vi "PCI-USB_ DO Notifier info.vi"(8 "error in":errorcluster, 10 "DO":T1) -> (0 "error out":errorcluster, 2 "Digital Output":bool[](array[boolean]), 3 "Update":bool)   [LabVIEW 2015]
uses:
  Digital out put.ctl
panel:
  in  "timeout in ms (-1)":i32=100
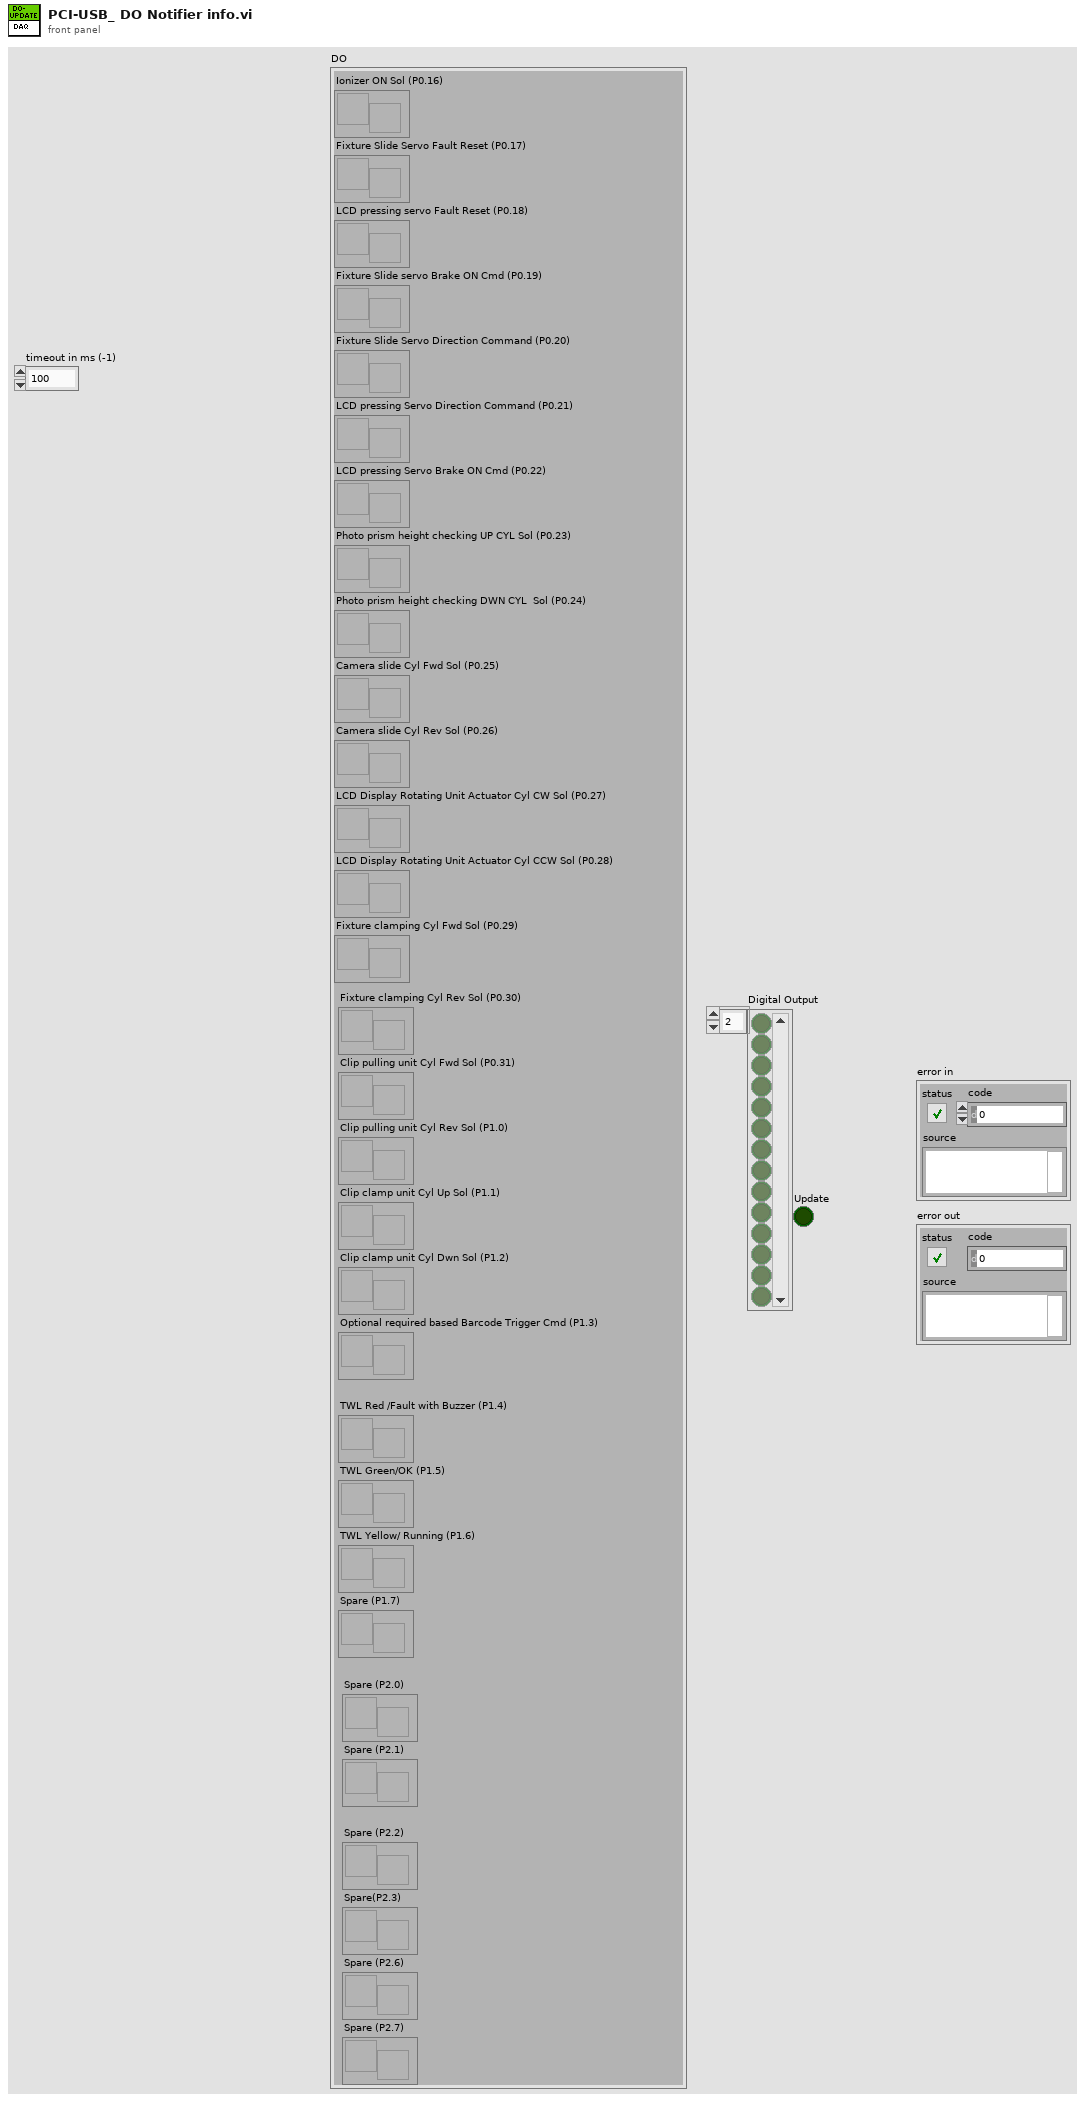
[diagram p1: front panel]
types:
  T1 = typedef "Digital out put.ctl" = cluster{"Ionizer ON Sol (P0.16)":refnum<notifier>, "Fixture Slide Servo Fault Reset (P0.17)":refnum<notifier>, "LCD pressing servo Fault Reset (P0.18)":refnum<notifier>, "Fixture Slide servo Brake ON Cmd (P0.19)":refnum<notifier>, "Fixture Slide Servo Direction Command (P0.20)":refnum<notifier>, "LCD pressing Servo Direction Command (P0.21)":refnum<notifier>, "LCD pressing Servo Brake ON Cmd (P0.22)":refnum<notifier>, "Photo prism height checking UP CYL Sol (P0.23)":refnum<notifier>, "Photo prism height checking DWN CYL  Sol (P0.24)":refnum<notifier>, "Camera slide Cyl Fwd Sol (P0.25)":refnum<notifier>, "Camera slide Cyl Rev Sol (P0.26)":refnum<notifier>, "LCD Display Rotating Unit Actuator Cyl CW Sol (P0.27)":refnum<notifier>, "LCD Display Rotating Unit Actuator Cyl CCW Sol (P0.28)":refnum<notifier>, "Fixture clamping Cyl Fwd Sol (P0.29)":refnum<notifier>, "Fixture clamping Cyl Rev Sol (P0.30)":refnum<notifier>, "Clip pulling unit Cyl Fwd Sol (P0.31)":refnum<notifier>, "Clip pulling unit Cyl Rev Sol (P1.0)":refnum<notifier>, "Clip clamp unit Cyl Up Sol (P1.1)":refnum<notifier>, "Clip clamp unit Cyl Dwn Sol (P1.2)":refnum<notifier>, "Optional required based Barcode Trigger Cmd (P1.3)":refnum<notifier>, "TWL Red /Fault with Buzzer (P1.4)":refnum<notifier>, "TWL Green/OK (P1.5)":refnum<notifier>, "TWL Yellow/ Running (P1.6)":refnum<notifier>, "Spare (P1.7)":refnum<notifier>, "Spare (P2.0)":refnum<notifier>, "Spare (P2.1)":refnum<notifier>, "Spare (P2.2)":refnum<notifier>, "Spare(P2.3)":refnum<notifier>, "Spare (P2.6)":refnum<notifier>, "Spare (P2.7) ":refnum<notifier>}
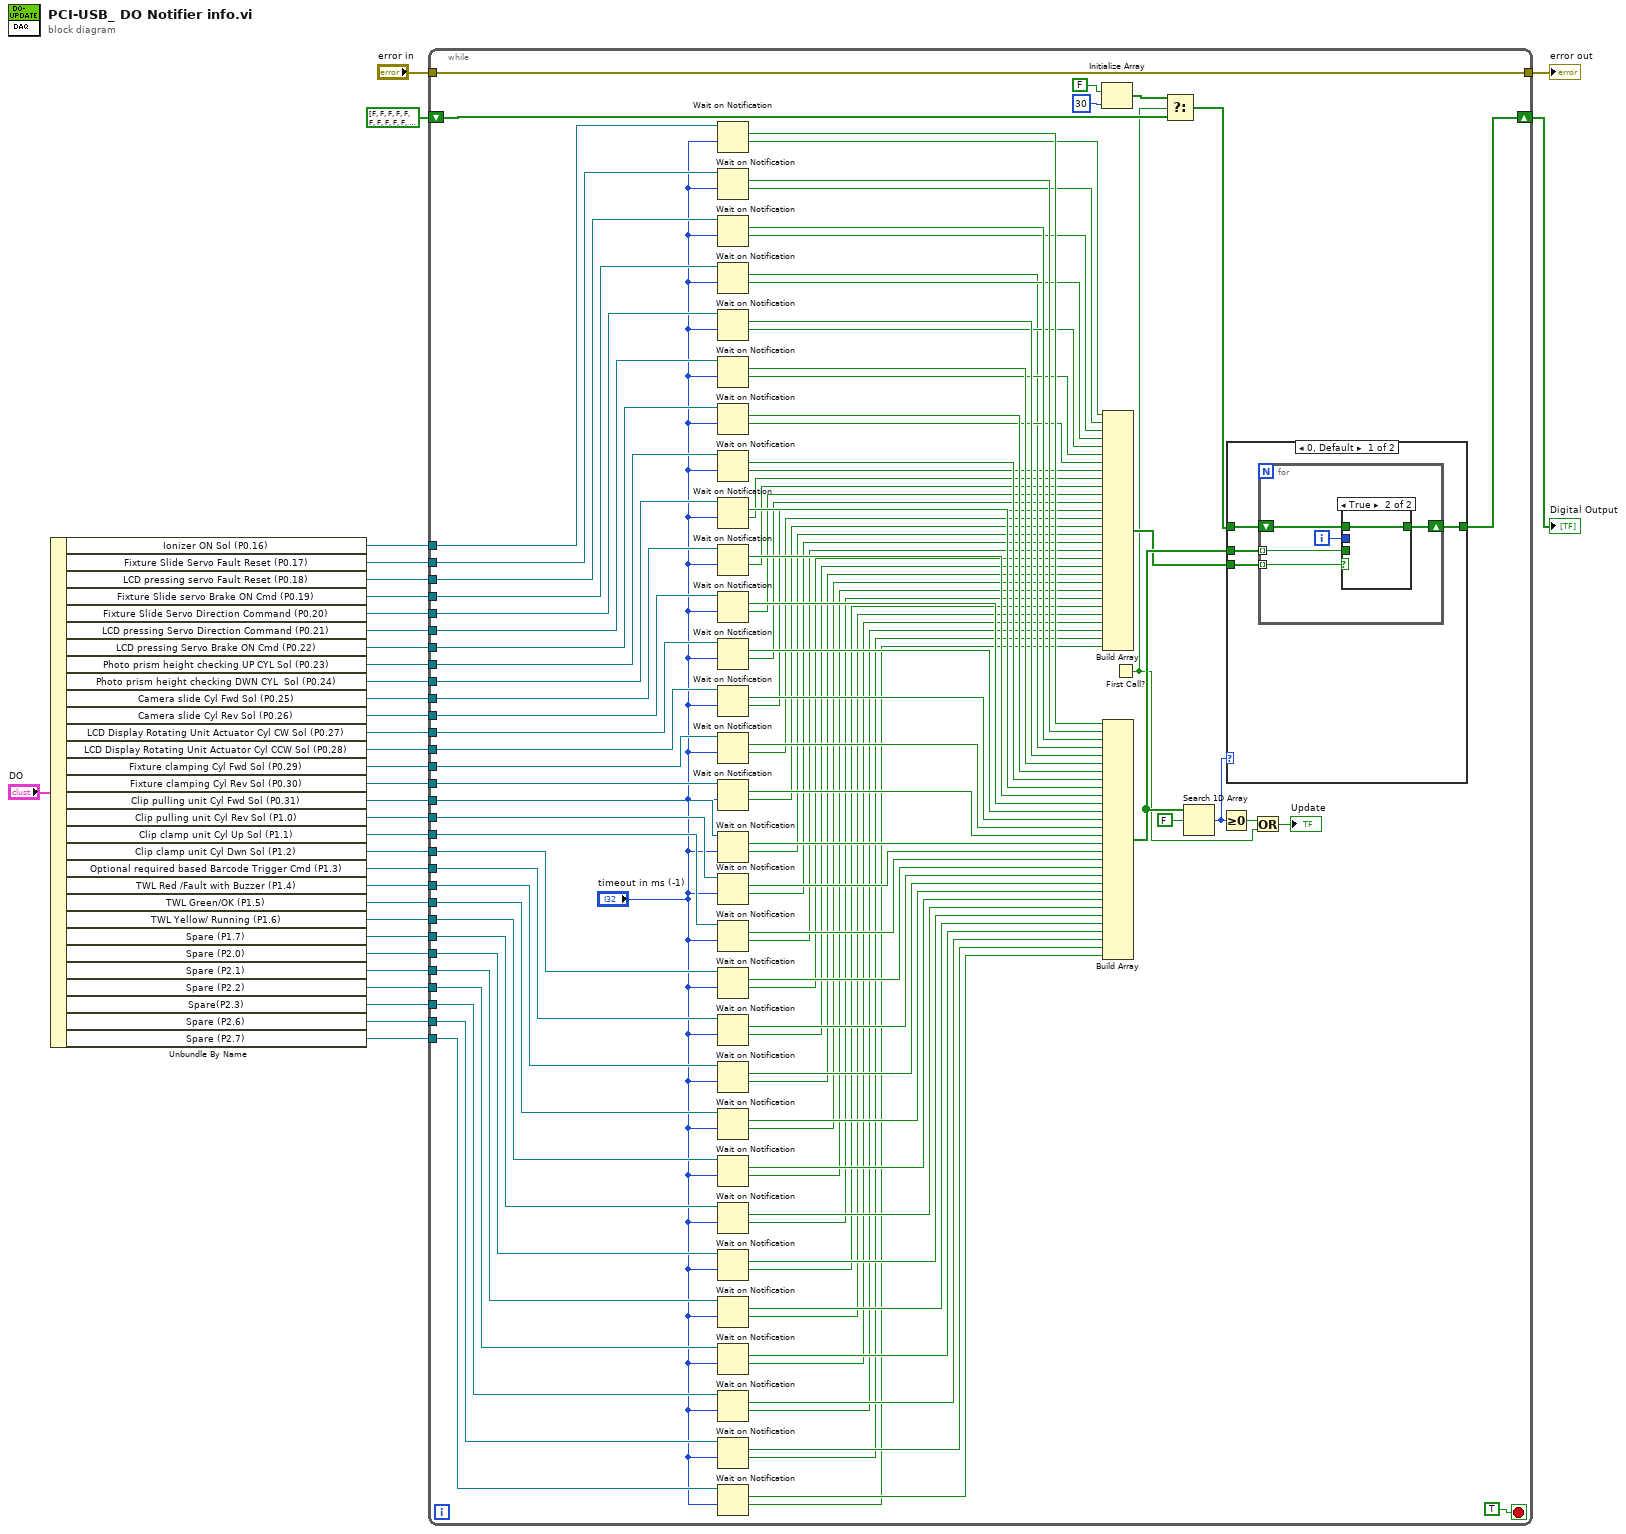
[diagram p0: block diagram]
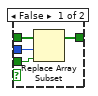
[diagram p2: hidden frame]
diagram:
  n1 = Unbundle By Name("DO") -> ("Ionizer ON Sol (P0.16)"=w35:refnum<notifier>, "Fixture Slide Servo Fault Reset (P0.17)"=w34:refnum<notifier>, "LCD pressing servo Fault Reset (P0.18)"=w33:refnum<notifier>, "Fixture Slide servo Brake ON Cmd (P0.19)"=w32:refnum<notifier>, "Fixture Slide Servo Direction Command (P0.20)"=w31:refnum<notifier>, "LCD pressing Servo Direction Command (P0.21)"=w30:refnum<notifier>, "LCD pressing Servo Brake ON Cmd (P0.22)"=w29:refnum<notifier>, "Photo prism height checking UP CYL Sol (P0.23)"=w25:refnum<notifier>, "Photo prism height checking DWN CYL  Sol (P0.24)"=w24:refnum<notifier>, "Camera slide Cyl Fwd Sol (P0.25)"=w23:refnum<notifier>, "Camera slide Cyl Rev Sol (P0.26)"=w22:refnum<notifier>, "LCD Display Rotating Unit Actuator Cyl CW Sol (P0.27)"=w21:refnum<notifier>, "LCD Display Rotating Unit Actuator Cyl CCW Sol (P0.28)"=w20:refnum<notifier>, "Fixture clamping Cyl Fwd Sol (P0.29)"=w18:refnum<notifier>, "Fixture clamping Cyl Rev Sol (P0.30)"=w17:refnum<notifier>, "Clip pulling unit Cyl Fwd Sol (P0.31)"=w16:refnum<notifier>, "Clip pulling unit Cyl Rev Sol (P1.0)"=w15:refnum<notifier>, "Clip clamp unit Cyl Up Sol (P1.1)"=w14:refnum<notifier>, "Clip clamp unit Cyl Dwn Sol (P1.2)"=w13:refnum<notifier>, "Optional required based Barcode Trigger Cmd (P1.3)"=w12:refnum<notifier>, "TWL Red /Fault with Buzzer (P1.4)"=w11:refnum<notifier>, "TWL Green/OK (P1.5)"=w10:refnum<notifier>, "TWL Yellow/ Running (P1.6)"=w9:refnum<notifier>, "Spare (P1.7)"=w8:refnum<notifier>, "Spare (P2.0)"=w7:refnum<notifier>, "Spare (P2.1)"=w6:refnum<notifier>, "Spare (P2.2)"=w5:refnum<notifier>, "Spare(P2.3)"=w4:refnum<notifier>, "Spare (P2.6)"=w3:refnum<notifier>, "Spare (P2.7)"=w2:refnum<notifier>)
  n2 = while {
    tunnel: w35 -> [w140]
    tunnel: w34 -> [w139]
    tunnel: w33 -> [w138]
    tunnel: w32 -> [w137]
    tunnel: w31 -> [w136]
    tunnel: w30 -> [w135]
    tunnel: w29 -> [w134]
    shift-right: [w117] -> w28
    shift-left: bool[] [FALSE, FALSE, FALSE, FALSE, FALSE, FALSE, FALSE, FALSE, FALSE, FALSE, FALSE, FALSE, FALSE, FALSE, FALSE, FALSE, FALSE, FALSE, FALSE, FALSE, FALSE, FALSE, FALSE, FALSE, FALSE, FALSE, FALSE, FALSE, FALSE, FALSE] -> [w115]
    tunnel: "error in" -> [w113]
    tunnel: [w113] -> w26
    tunnel: w25 -> [w108]
    tunnel: w24 -> [w107]
    tunnel: w23 -> [w106]
    tunnel: w22 -> [w105]
    tunnel: w21 -> [w104]
    tunnel: w20 -> [w103]
    tunnel: w18 -> [w90]
    tunnel: w17 -> [w84]
    tunnel: w16 -> [w83]
    tunnel: w15 -> [w82]
    tunnel: w14 -> [w81]
    tunnel: w13 -> [w80]
    tunnel: w12 -> [w79]
    tunnel: w11 -> [w78]
    tunnel: w10 -> [w77]
    tunnel: w9 -> [w76]
    tunnel: w8 -> [w75]
    tunnel: w7 -> [w74]
    tunnel: w6 -> [w73]
    tunnel: w5 -> [w72]
    tunnel: w4 -> [w71]
    tunnel: w3 -> [w70]
    tunnel: w2 -> [w69]
    stop <- TRUE stop-if-true
    n3 = Wait on Notification(notifier=w140, timeout in ms (-1)="timeout in ms (-1)") -> (notification=w133:bool, timed out?=w127:bool)  [unwired: 2 in, 2 out]
    n4 = Wait on Notification(notifier=w139, timeout in ms (-1)="timeout in ms (-1)") -> (notification=w132:bool, timed out?=w126:bool)  [unwired: 2 in, 2 out]
    n5 = Wait on Notification(notifier=w138, timeout in ms (-1)="timeout in ms (-1)") -> (notification=w131:bool, timed out?=w125:bool)  [unwired: 2 in, 2 out]
    n6 = Wait on Notification(notifier=w137, timeout in ms (-1)="timeout in ms (-1)") -> (notification=w114:bool, timed out?=w124:bool)  [unwired: 2 in, 2 out]
    n7 = Wait on Notification(notifier=w136, timeout in ms (-1)="timeout in ms (-1)") -> (notification=w130:bool, timed out?=w123:bool)  [unwired: 2 in, 2 out]
    n8 = Wait on Notification(notifier=w135, timeout in ms (-1)="timeout in ms (-1)") -> (notification=w129:bool, timed out?=w122:bool)  [unwired: 2 in, 2 out]
    n9 = Wait on Notification(notifier=w134, timeout in ms (-1)="timeout in ms (-1)") -> (notification=w128:bool, timed out?=w121:bool)  [unwired: 2 in, 2 out]
    n10 = Wait on Notification(notifier=w108, timeout in ms (-1)="timeout in ms (-1)") -> (notification=w102:bool, timed out?=w96:bool)  [unwired: 2 in, 2 out]
    n11 = Wait on Notification(notifier=w107, timeout in ms (-1)="timeout in ms (-1)") -> (notification=w101:bool, timed out?=w95:bool)  [unwired: 2 in, 2 out]
    n12 = Wait on Notification(notifier=w106, timeout in ms (-1)="timeout in ms (-1)") -> (notification=w100:bool, timed out?=w94:bool)  [unwired: 2 in, 2 out]
    n13 = Wait on Notification(notifier=w105, timeout in ms (-1)="timeout in ms (-1)") -> (notification=w99:bool, timed out?=w93:bool)  [unwired: 2 in, 2 out]
    n14 = Wait on Notification(notifier=w104, timeout in ms (-1)="timeout in ms (-1)") -> (notification=w98:bool, timed out?=w92:bool)  [unwired: 2 in, 2 out]
    n15 = Wait on Notification(notifier=w103, timeout in ms (-1)="timeout in ms (-1)") -> (notification=w97:bool, timed out?=w91:bool)  [unwired: 2 in, 2 out]
    n16 = Wait on Notification(notifier=w90, timeout in ms (-1)="timeout in ms (-1)") -> (notification=w89:bool, timed out?=w88:bool)  [unwired: 2 in, 2 out]
    n17 = Wait on Notification(notifier=w84, timeout in ms (-1)="timeout in ms (-1)") -> (notification=w67:bool, timed out?=w66:bool)  [unwired: 2 in, 2 out]
    n18 = Wait on Notification(notifier=w83, timeout in ms (-1)="timeout in ms (-1)") -> (notification=w65:bool, timed out?=w64:bool)  [unwired: 2 in, 2 out]
    n19 = Wait on Notification(notifier=w82, timeout in ms (-1)="timeout in ms (-1)") -> (notification=w63:bool, timed out?=w62:bool)  [unwired: 2 in, 2 out]
    n20 = Wait on Notification(notifier=w81, timeout in ms (-1)="timeout in ms (-1)") -> (notification=w61:bool, timed out?=w60:bool)  [unwired: 2 in, 2 out]
    n21 = Wait on Notification(notifier=w80, timeout in ms (-1)="timeout in ms (-1)") -> (notification=w59:bool, timed out?=w58:bool)  [unwired: 2 in, 2 out]
    n22 = Wait on Notification(notifier=w79, timeout in ms (-1)="timeout in ms (-1)") -> (notification=w57:bool, timed out?=w56:bool)  [unwired: 2 in, 2 out]
    n23 = Wait on Notification(notifier=w78, timeout in ms (-1)="timeout in ms (-1)") -> (notification=w55:bool, timed out?=w54:bool)  [unwired: 2 in, 2 out]
    n24 = Wait on Notification(notifier=w77, timeout in ms (-1)="timeout in ms (-1)") -> (notification=w53:bool, timed out?=w52:bool)  [unwired: 2 in, 2 out]
    n25 = Wait on Notification(notifier=w76, timeout in ms (-1)="timeout in ms (-1)") -> (notification=w51:bool, timed out?=w50:bool)  [unwired: 2 in, 2 out]
    n26 = Wait on Notification(notifier=w75, timeout in ms (-1)="timeout in ms (-1)") -> (notification=w49:bool, timed out?=w48:bool)  [unwired: 2 in, 2 out]
    n27 = Wait on Notification(notifier=w74, timeout in ms (-1)="timeout in ms (-1)") -> (notification=w47:bool, timed out?=w46:bool)  [unwired: 2 in, 2 out]
    n28 = Wait on Notification(notifier=w73, timeout in ms (-1)="timeout in ms (-1)") -> (notification=w45:bool, timed out?=w44:bool)  [unwired: 2 in, 2 out]
    n29 = Wait on Notification(notifier=w72, timeout in ms (-1)="timeout in ms (-1)") -> (notification=w43:bool, timed out?=w42:bool)  [unwired: 2 in, 2 out]
    n30 = Wait on Notification(notifier=w71, timeout in ms (-1)="timeout in ms (-1)") -> (notification=w41:bool, timed out?=w40:bool)  [unwired: 2 in, 2 out]
    n31 = Wait on Notification(notifier=w70, timeout in ms (-1)="timeout in ms (-1)") -> (notification=w39:bool, timed out?=w38:bool)  [unwired: 2 in, 2 out]
    n32 = Wait on Notification(notifier=w69, timeout in ms (-1)="timeout in ms (-1)") -> (notification=w37:bool, timed out?=w36:bool)  [unwired: 2 in, 2 out]
    n33 = Initialize Array(FALSE, 30 ("dimension size")) -> (w85:bool[])
    n34 = Build Array(w127, w126, w125, w124, w123, w122, w121, w96, w95, w94, w93, w92, w91, w88, w66, w64, w62, w60, w58, w56, w54, w52, w50, w48, w46, w44, w42, w40, w38, w36) -> (w118:bool[])
    n35 = Build Array(w133, w132, w131, w114, w130, w129, w128, w102, w101, w100, w99, w98, w97, w89, w67, w65, w63, w61, w59, w57, w55, w53, w51, w49, w47, w45, w43, w41, w39, w37) -> (w119:bool[])
    n36 = First Call?() -> (First Call?: T/F=w110:bool)
    n37 = Select(t=w85, s=w110, f=w115) -> (s? t:f=w116:bool[])
    n38 = Search 1D Array(1D array=w119, element=FALSE) -> (index of element=w111:i32)  [unwired: 1 in]
    n39 = Greater Or Equal To 0?(x=w111) -> (x >= 0?=w112:bool)
    n40 = case shown="0, Default" w111 {
      tunnel: w119 -> [w145 _]
      tunnel: w118 -> [w144 _]
      tunnel: w116 -> [w143 w156]
      tunnel: [w142 w156] -> w117
      frame 0, Default {
        n41 = for {
          tunnel: w145 -> [w149] mode=indexing
          tunnel: w144 -> [w150] mode=indexing
          shift-right: [w146] -> w142
          shift-left: w143 -> [w147]
          i -> [w148]
          n42 = case shown="True" w150 {
            tunnel: w149 -> [w152 _]
            tunnel: w148 -> [w153 _]
            tunnel: w147 -> [w154 w155]
            tunnel: [w151 w155] -> w146
            frame False {
              n43 = Replace Array Subset(array=w154, new element=w152, index=w153) -> (w151:bool[])
            }
            frame True {
            }
          }
        }
      }
      frame -1 {
      }
    }
    n44 = Or(x=w112, y=w110) -> (x .or. y?=→"Update":bool)
  }
  "Digital Output" <- w28
  "error out" <- w26
